vi "crop_rectangular.vi"(10 "dbl_ar_crop_correction":dbl[](array[numeric])=[0.0, 0.0, 0.0, 0.0], 11 "image_in":T1) -> (2 "crop boundaries":dbl[](array[numeric]), 3 "cropped image out":T1)   [LabVIEW 2011]
uses:
  <vilib>/vision/Image Controls.llb/IMAQ Image.ctl
  global_vars.vi
  <vilib>/vision/NI_Vision_Development_Module.lvlib
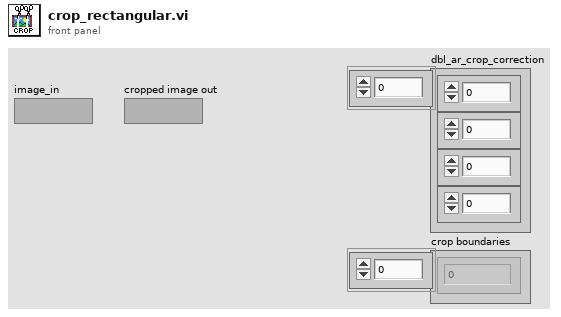
[diagram p1: front panel]
types:
  T1 = typedef "IMAQ Image.ctl" = refnum<image>
  T2 = typedef "Image Type" = u32
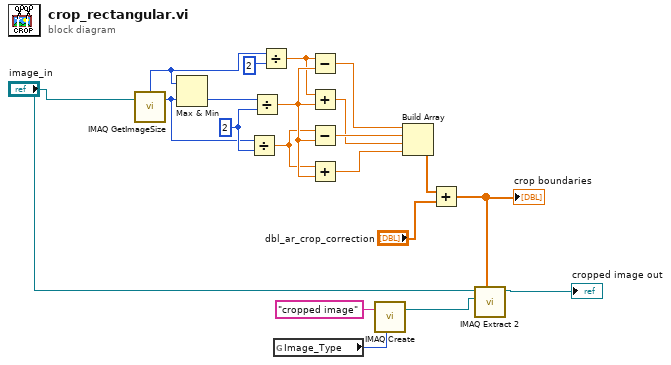
[diagram p0: block diagram]
diagram:
  w18 = 2 ("y")
  n1 = call "IMAQ GetImageSize"("Image"="image_in") -> ("Y Resolution"=w10:i32, "X Resolution"=w8:i32)  [unwired: 3 in, 1 out]
  n2 = Max & Min(x=w8, y=w10) -> (min(x,y)=w17:i32)  [unwired: 1 out]
  n3 = Divide(x=w10, y=w18) -> (x/y=w12:dbl)
  n4 = Divide(x=w17, y=w18) -> (x/y=w16:dbl)
  n5 = Divide(x=w8, y=2) -> (x/y=w11:dbl)
  n6 = global read "global_vars.vi" "Image_Type"() -> (w5:T2)
  n7 = Subtract(x=w11, y=w16) -> (x-y=w13:dbl)
  n8 = Add(x=w11, y=w16) -> (x+y=w14:dbl)
  n9 = Subtract(x=w12, y=w16) -> (x-y=w20:dbl)
  n10 = Add(x=w12, y=w16) -> (x+y=w19:dbl)
  n11 = call "IMAQ Create"("Image Name"="cropped image", "Image Type"=w5) -> ("New Image"=w6:T1)  [unwired: 2 in, 2 out]
  n12 = Build Array(w13, w20, w14, w19) -> (w2:dbl[])
  n13 = Add(x=w2, y="dbl_ar_crop_correction") -> (x+y=w3:dbl[])
  "crop boundaries" <- w3
  n14 = call "IMAQ Extract 2"("Optional Rectangle"=w3, "Image Dst"=w6, "Image Src"="image_in") -> ("Image Dst Out"=→"cropped image out":T1)  [unwired: 7 in, 1 out]
